vi "Slice Module.vi"(8 "Error In":errorcluster, 10 "Table Stages":T3, 11 "Vibratome":T4={"Z Bottom [mm]"=0.0, "Pre Cut Dwell [s]"=0.0, "Blade Frequency [RPM]"=0, "Slice Speed [mm/s]"=0.0, "Post Cut Dwell [s]"=0.0, "Ramp Time [s]"=0.0, "Start X [mm]"=0.0, "Start Y [mm]"=0.0, "Slice Length [mm]"=0.0, "Axis"=enum."X Axis", "Controller VISA Ref"="COM4"}) -> (0 "Error Out":errorcluster, 2 "Abort":bool, 3 "Finished":bool)   [LabVIEW 2014]
uses:
  Hardware/Table Stage/Controls/Translation Stage Cluster.ctl
  Controls/Translation Stage Types.ctl
  Controls/QueueNames.ctl
  Controls/Queue Manager Actions.ctl
  Hardware/Table Stage/Controls/Motion Translation Module Control.ctl
  Controls/Set Get Controls.ctl
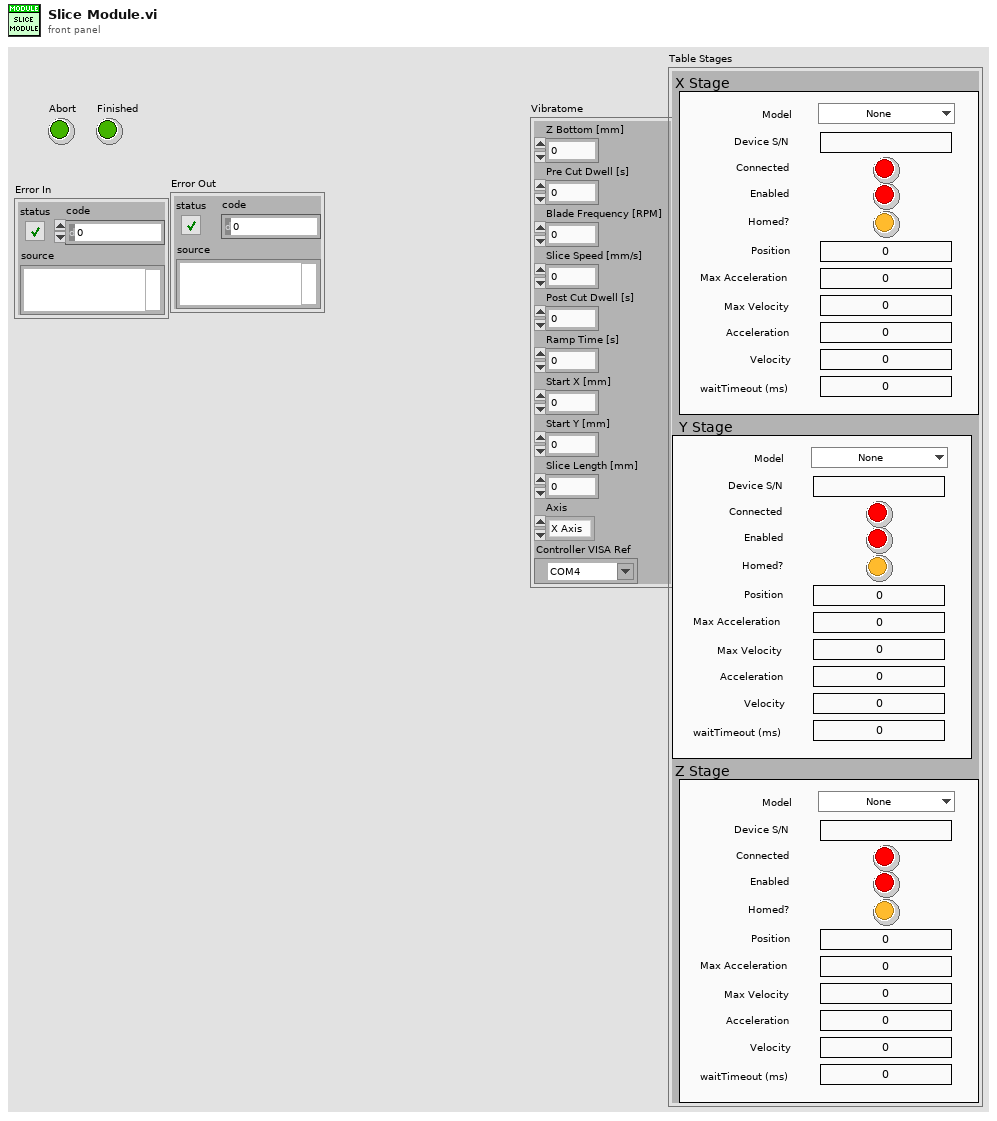
[diagram p1: front panel]
types:
  T1 = typedef "Translation Stage Cluster.ctl" = cluster{"Position":dbl, "Is.Enabled?":bool, "Is.Connected?":bool, "Device SN":string, "AccelerationMaximum":dbl, "VelocityMaximum":dbl, "Acceleration":dbl, "Velocity":dbl, "waitTimeout (ms)":i32, "Model":T2, "Is.Homed?":bool}
  T2 = typedef "Translation Stage Types.ctl" = enum16{"None", "Thorlabs LTS", "Thorlabs MLJ"}
  T3 = cluster{"X Stage":T1, "Y Stage":T1, "Z Stage":T1}
  T4 = cluster{"Z Bottom [mm]":dbl, "Pre Cut Dwell [s]":dbl, "Blade Frequency [RPM]":u16, "Slice Speed [mm/s]":dbl, "Post Cut Dwell [s]":dbl, "Ramp Time [s]":dbl, "Start X [mm]":dbl, "Start Y [mm]":dbl, "Slice Length [mm]":dbl, "Axis":enum16{"X Axis", "Y Axis", "Z Axis"}, "Controller VISA Ref":refnum<visa-resource-name>}
  T5 = typedef "Set Get Controls.ctl" = enum16{"Set", "Get"}
  T6 = typedef "Motion Translation Module Control.ctl" = enum16{"Init", "Home", "Status", "Velocity/Accel", "Position", "Jog", "Stop", "Uninit", "Enable", "Disable"}
  T7 = cluster{"Source for Velocity":enum16{"Interface", "Voltage (AI)", "PWM (AI)", "Current Target (AI)", "Current Target w/ Preset (AI)"}, "Mode":enum16{"Continuous", "Stepper Motor", "Analog Position Ctrl", "Encoder"}, "Target Velocity [RPM]":i16}
  T8 = enum16{"Set Configuration", "Get Configuration", "Enable Motor", "Disable Motor", "Get Status", "Open Session", "Close Session", "Set Limits", "Get Limits"}
  T9 = typedef "Queue Manager Actions.ctl" = enum16{"Init", "Enqueue", "Enqueue All", "Preview Queue", "Dequeue", "Get Status", "Flush Queue", "Flush All Queues", "Release All Queues", "Release Queue", "Enqueue at Opposite End"}
  T10 = typedef "QueueNames.ctl" = enum16{"Main GUI", "Main Scan Processor", "Main Display", "Main Table Stage GUI", "Main Table Stage Proc.", "Scan Engine", "Vibratome GUI", "Vibratome Processor", "Slice Engine"}
  T11 = typedef "MessagePacket.ctl" = cluster{"Message":string, "Parameter":variant}
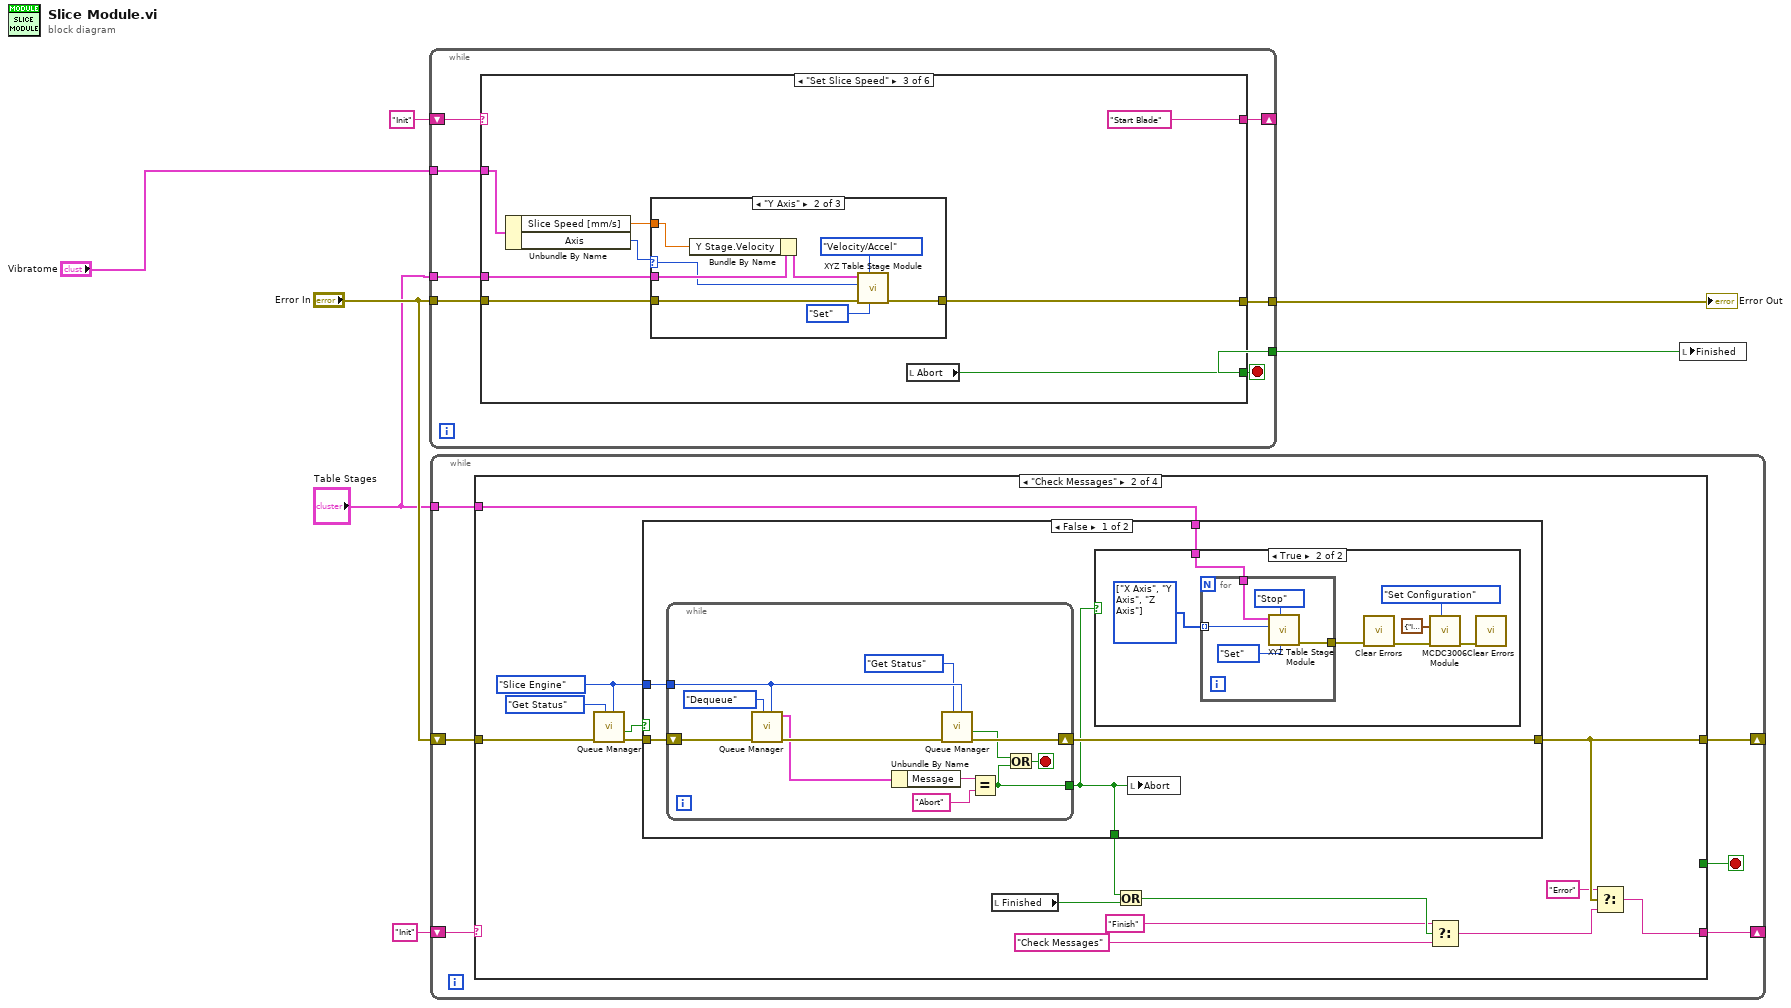
[diagram p0: block diagram]
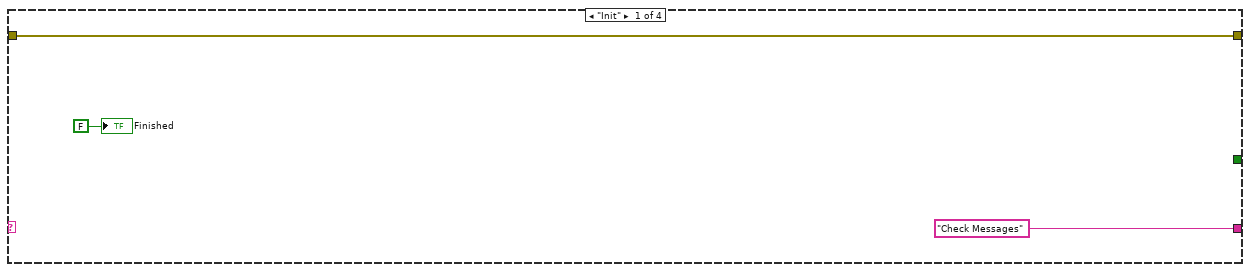
[diagram p2: hidden frame]
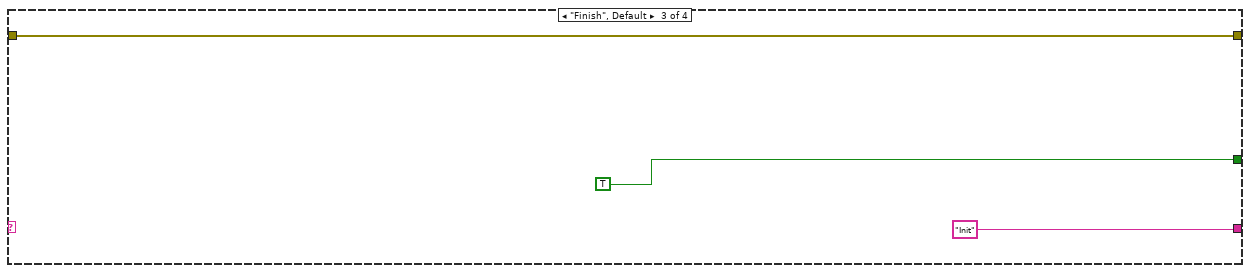
[diagram p5: hidden frame]
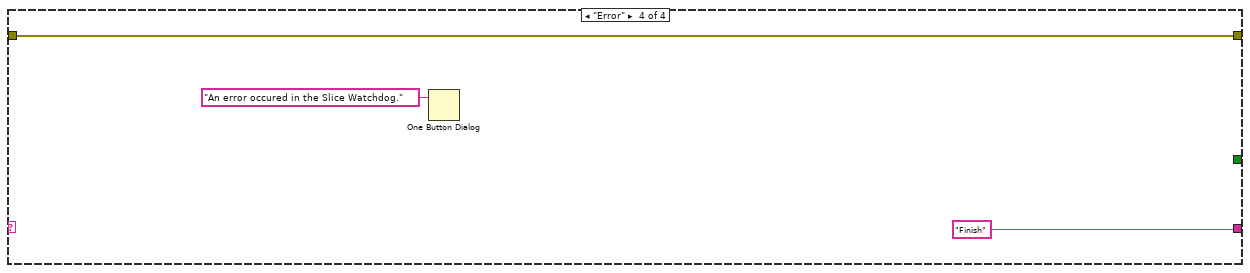
[diagram p6: hidden frame]
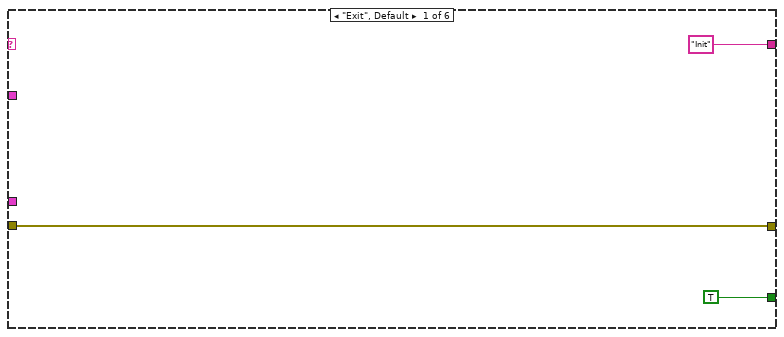
[diagram p7: hidden frame]
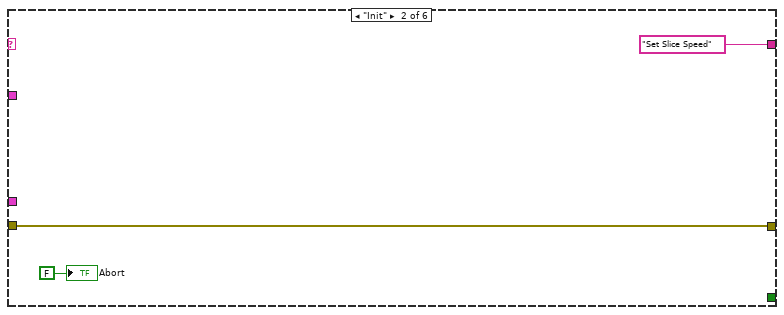
[diagram p8: hidden frame]
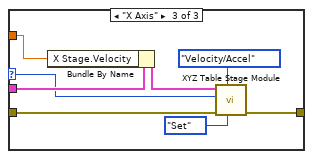
[diagram p10: hidden frame]
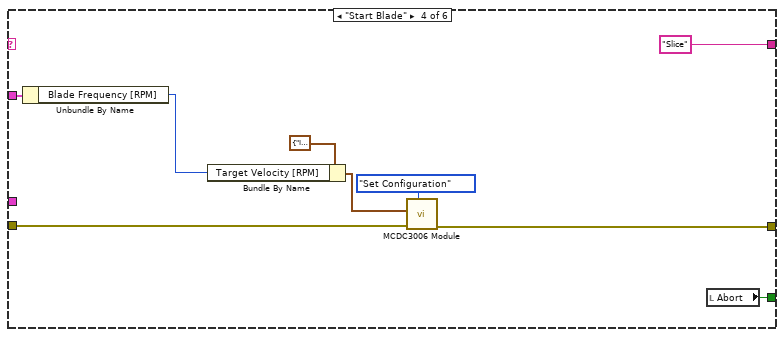
[diagram p11: hidden frame]
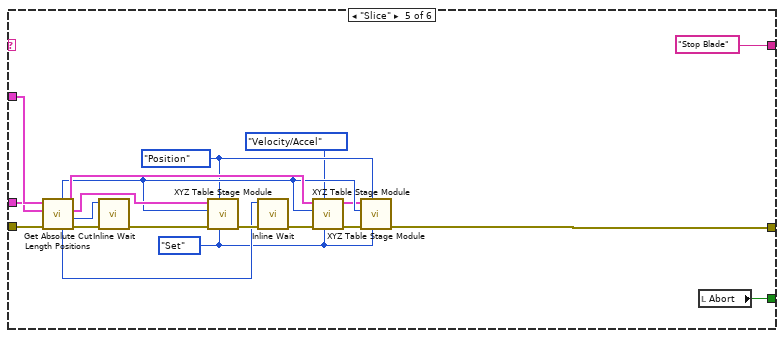
[diagram p12: hidden frame]
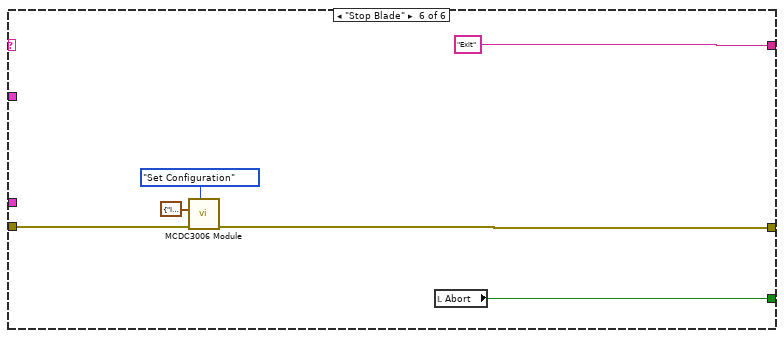
[diagram p13: hidden frame]
diagram:
  n1 = while {
    shift-right: [w13] -> _
    shift-left: "Init" -> [w14]
    tunnel: "Error In" -> [w12]
    tunnel: "Table Stages" -> [w11]
    tunnel: "Vibratome" -> [w10]
    tunnel: [w9] -> w5
    tunnel: [w8] -> w3
    stop <- w8 stop-if-true
    n2 = case shown="\"Set Slice Speed\"" w14 {
      tunnel: ["Init" "Set Slice Speed" "Start Blade" "Slice" "Stop Blade" "Exit"] -> w13
      tunnel: [TRUE _ w27 w53 w73 w79] -> w8
      tunnel: w12 -> [w15 w18 w26 w52 w71 w76]
      tunnel: w11 -> [_ _ w24 _ w70 _]
      tunnel: w10 -> [_ _ w23 w50 w72 _]
      tunnel: [w15 w18 w25 w46 w60 w75] -> w9
      frame "Exit", Default {
      }
      frame "Init" {
        "Abort" <- FALSE ("Abort")
      }
      frame "Set Slice Speed" {
        n3 = Unbundle By Name(w23) -> ("Slice Speed [mm/s]"=w22:dbl, "Axis"=w21:enum16{"X Axis", "Y Axis", "Z Axis"})
        n4 = case shown="\"Y Axis\"" w21 {
          selector: w21 -> [_ w32 w40]
          tunnel: w26 -> [w29 w37 w45]
          tunnel: [w29 w36 w44] -> w25
          tunnel: w24 -> [_ w35 w43]
          tunnel: w22 -> [_ w31 w39]
          frame "Z Axis", Default {
          }
          frame "Y Axis" {
            n5 = Bundle By Name(cluster=w35, "Y Stage.Velocity"=w31) -> (w33:T3)
            n6 = call "XYZ Table Stage Module.vi"("Set/Get"=Set_Get_Controls."Set", "Action"=Motion_Translation_Module_Control."Velocity/Accel", "Error In"=w37, "Axis"=w32, "Table Stages"=w33) -> ("Error Out"=w36:errorcluster)  [unwired: 5 in, 1 out]
          }
          frame "X Axis" {
            n7 = Bundle By Name(cluster=w43, "X Stage.Velocity"=w39) -> (w41:T3)
            n8 = call "XYZ Table Stage Module.vi"("Set/Get"=Set_Get_Controls."Set", "Action"=Motion_Translation_Module_Control."Velocity/Accel", "Error In"=w45, "Axis"=w40, "Table Stages"=w41) -> ("Error Out"=w44:errorcluster)  [unwired: 5 in, 1 out]
          }
        }
        n9 = local read "Abort"() -> (w27:bool)
      }
      frame "Start Blade" {
        n10 = Unbundle By Name(w50) -> ("Blade Frequency [RPM]"=w48:u16)
        n11 = Bundle By Name(cluster=T7 {"Source for Velocity"=enum."Interface", "Mode"=enum."Continuous", "Target Velocity [RPM]"=0} ("Configuration [In]"), "Target Velocity [RPM]"=w48) -> (w49:T7)
        n12 = call "MCDC3006 Module.vi"("Actions"=T8."Set Configuration", "Error In"=w52, "Configuration [In]"=w49) -> ("Error Out"=w46:errorcluster)  [unwired: 4 in, 4 out]
        n13 = local read "Abort"() -> (w53:bool)
      }
      frame "Slice" {
        w57 = Motion_Translation_Module_Control."Position" ("Action")
        w59 = Set_Get_Controls."Set" ("Set/Get")
        n14 = call "Get Absolute Cut Length Positions.vi"("error in (no error)"=w71, "Table Stages"=w70, "Vibratome"=w72) -> ("error out"=w69:errorcluster, "Pre Cut Dwell [s]"=w63:u32, "Slice Position"=w68:T3, "Original Position"=w61:T3, "Post Cut Dwell [s]"=w65:u32, "Slice Axis"=w58:enum16{"X Axis", "Y Axis", "Z Axis"})  [unwired: 3 in]
        n15 = call "Inline Wait.vi"("Error In"=w69, "milliseconds to wait"=w63) -> ("Error Out"=w64:errorcluster)  [unwired: 9 in]
        n16 = call "XYZ Table Stage Module.vi"("Set/Get"=w59, "Action"=w57, "Error In"=w64, "Axis"=w58, "Table Stages"=w68) -> ("Error Out"=w67:errorcluster)  [unwired: 5 in, 1 out]
        n17 = call "Inline Wait.vi"("Error In"=w67, "milliseconds to wait"=w65) -> ("Error Out"=w66:errorcluster)  [unwired: 9 in]
        n18 = call "XYZ Table Stage Module.vi"("Set/Get"=w59, "Action"=Motion_Translation_Module_Control."Velocity/Accel", "Error In"=w66, "Axis"=w58, "Table Stages"=w61) -> ("Error Out"=w62:errorcluster, "Table Stages Out"=w55:T3)  [unwired: 5 in]
        n19 = call "XYZ Table Stage Module.vi"("Set/Get"=w59, "Action"=w57, "Error In"=w62, "Axis"=w58, "Table Stages"=w55) -> ("Error Out"=w60:errorcluster)  [unwired: 5 in, 1 out]
        n20 = local read "Abort"() -> (w73:bool)
      }
      frame "Stop Blade" {
        n21 = call "MCDC3006 Module.vi"("Actions"=T8."Set Configuration", "Error In"=w76, "Configuration [In]"=T7 {"Source for Velocity"=enum."Interface", "Mode"=enum."Continuous", "Target Velocity [RPM]"=0}) -> ("Error Out"=w75:errorcluster)  [unwired: 4 in, 4 out]
        n22 = local read "Abort"() -> (w79:bool)
      }
    }
  }
  "Error Out" <- w5
  n23 = while {
    shift-right: [w85] -> _
    shift-left: "Init" -> [w86]
    shift-right: [w84] -> _
    shift-left: "Error In" -> [w83]
    tunnel: "Table Stages" -> [w81]
    stop <- w82 stop-if-true
    n24 = case shown="\"Check Messages\"" w86 {
      tunnel: ["Check Messages" w93 "Init" "Finish"] -> w85
      tunnel: [w87 w92 w137 w140] -> w84
      tunnel: w83 -> [w87 w100 w137 w140]
      tunnel: [_ _ TRUE ("Abort") _] -> w82
      tunnel: w81 -> [_ w90 _ _]
      frame "Init" {
        "Finished" <- FALSE ("Abort")
      }
      frame "Check Messages" {
        w101 = QueueNames."Slice Engine" ("Queue Name")
        n25 = call "Queue Manager.vi"("Queue Name"=w101, "Action"=Queue_Manager_Actions."Get Status", "Error In"=w100) -> ("Error Out"=w102:errorcluster, "Empty?"=w103:bool)  [unwired: 6 in, 1 out]
        n26 = case shown="False" w103 {
          tunnel: w102 -> [w109 w134]
          tunnel: w101 -> [w108 _]
          tunnel: [w107 w134] -> w92
          tunnel: [w106 _] -> w99
          tunnel: w90 -> [w105 _]
          frame False {
            n27 = while {
              tunnel: w108 -> [w129]
              shift-right: [w130] -> w107
              shift-left: w109 -> [w133]
              tunnel: [w122] -> w106
              stop <- w123 stop-if-true
              n28 = call "Queue Manager.vi"("Queue Name"=w129, "Action"=Queue_Manager_Actions."Dequeue", "Error In"=w133) -> ("Error Out"=w131:errorcluster, "Message Packet [Out]"=w127:T11)  [unwired: 6 in, 1 out]
              n29 = Unbundle By Name(w127) -> ("Message"=w126:string)
              n30 = call "Queue Manager.vi"("Queue Name"=w129, "Action"=Queue_Manager_Actions."Get Status", "Error In"=w131) -> ("Error Out"=w130:errorcluster, "Empty?"=w124:bool)  [unwired: 6 in, 1 out]
              n31 = Equal?(x=w126, y="Abort") -> (x = y?=w122:bool)
              n32 = Or(x=w124, y=w122) -> (x .or. y?=w123:bool)
            }
            n33 = case shown="True" w106 {
              tunnel: w105 -> [_ w115]
              frame False {
              }
              frame True {
                w110 = enum16{"X Axis", "Y Axis", "Z Axis"}[] [enum."X Axis", enum."Y Axis", enum."Z Axis"] items=["X Axis", "Y Axis", "Z Axis"]
                n34 = for {
                  tunnel: [w121] -> w116
                  tunnel: w115 -> [w119]
                  tunnel: w110 -> [w117] mode=indexing
                  n35 = call "XYZ Table Stage Module.vi"("Set/Get"=Set_Get_Controls."Set", "Action"=Motion_Translation_Module_Control."Stop", "Axis"=w117, "Table Stages"=w119) -> ("Error Out"=w121:errorcluster)  [unwired: 6 in, 1 out]
                }
                n36 = call <vilib>:"Clear Errors.vi"("error in (no error)"=w116) -> ("error out"=w114:errorcluster)  [unwired: 5 in, 1 out]
                n37 = call "MCDC3006 Module.vi"("Actions"=T8."Set Configuration", "Error In"=w114, "Configuration [In]"=T7 {"Source for Velocity"=enum."Interface", "Mode"=enum."Continuous", "Target Velocity [RPM]"=0}) -> ("Error Out"=w111:errorcluster)  [unwired: 4 in, 4 out]
                n38 = call <vilib>:"Clear Errors.vi"("error in (no error)"=w111) -> ()  [unwired: 5 in, 2 out]
              }
            }
            n39 = local write "Abort"(w106) -> ()
          }
          frame True {
          }
        }
        n40 = local read "Finished"() -> (w98:bool)
        n41 = Or(x=w99, y=w98) -> (x .or. y?=w96:bool)
        n42 = Select(t="Finish", s=w96, f="Check Messages") -> (s? t:f=w94:string)
        n43 = Select(t="Error", s=w92, f=w94) -> (s? t:f=w93:string)
      }
      frame "Finish", Default {
      }
      frame "Error" {
        n44 = One Button Dialog(message="An error occured in the Slice Watchdog.") -> ()  [unwired: 1 in, 1 out]
      }
    }
  }
  n45 = local write "Finished"(w3) -> ()
